vi "Create Client.vi"(8 "error in (no error)":errorcluster, 10 "certificatePath":string, 11 "address":string) -> (0 "error out":errorcluster, 3 "Client Ref Out":T1)   [LabVIEW 2019, in "gprc-lvsupport.lvlib"]
uses:
  gprc-lvsupport.lvlib
  Server API/typeDefs/grpcId.ctl
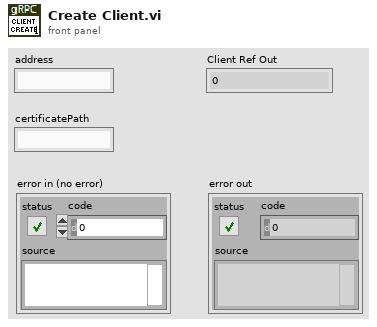
[diagram p1: front panel]
types:
  T1 = typedef "gprc-lvsupport.lvlib/grpcId.ctl" = u64
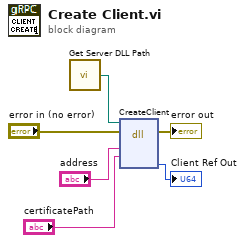
[diagram p0: block diagram]
diagram:
  n1 = call "Get Server DLL Path.vi"() -> ("Server dll path"=w5:path)
  n2 = dll-call lib="?" fn="CreateClient"(path in=w5, error in="error in (no error)", "address"="address", "certificatePath"="certificatePath") -> (error out=→"error out":errorcluster, "clientId"=→"Client Ref Out":u64)  [unwired: 5 in, 1 out]
